vi "Test.vi"() -> ()   [LabVIEW 2015, in "SLSC Switch.lvlib" / "slscsl.lvclass"]
uses:
  slscsl.lvclass
  SwitchActionsArray.ctl
  SwitchAction.ctl
  RelayAction.ctl
panel:
  out "Relays":T1 {"RelayAction" items=["CloseRelay"=21, "OpenRelay"=20]}
  out "Disconnect":T1 {"RelayAction" items=["CloseRelay"=21, "OpenRelay"=20]}
  out "Connect":T1 {"RelayAction" items=["CloseRelay"=21, "OpenRelay"=20]}
  in  "error in (no error)":errorcluster
  out "error out":errorcluster
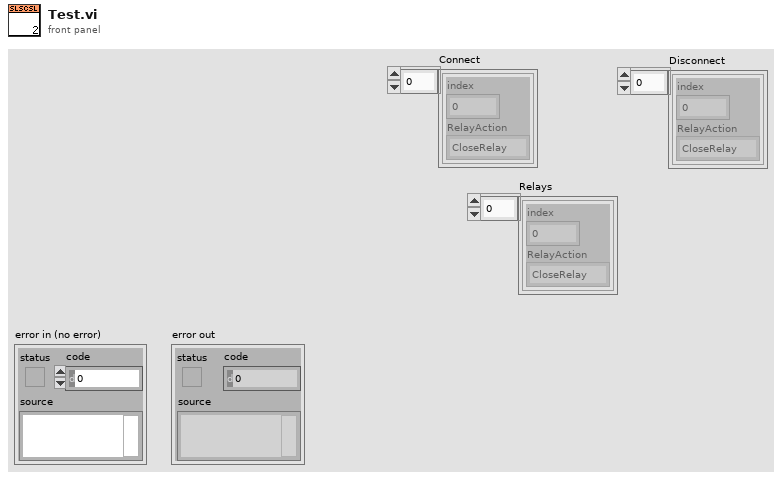
[diagram p1: front panel]
types:
  T1 = typedef "SLSC Switch.lvlib/slscsl.lvclass/SwitchActionsArray.ctl" = T2[]
  T2 = typedef "SLSC Switch.lvlib/slscsl.lvclass/SwitchAction.ctl" = cluster{"index":i32, "RelayAction":T3}
  T3 = typedef "SLSC Switch.lvlib/slscsl.lvclass/RelayAction.ctl" = u32
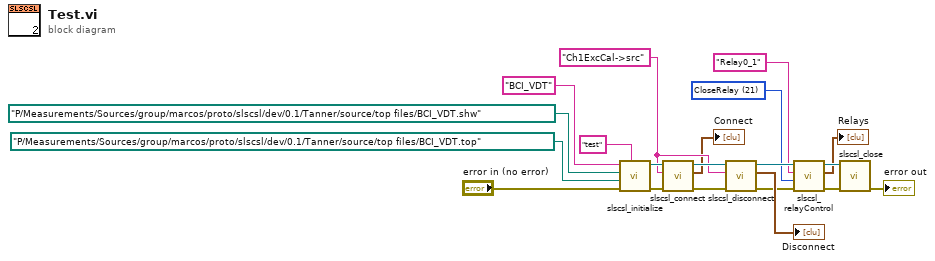
[diagram p0: block diagram]
diagram:
  w2 = T3 21 items=["CloseRelay"=21, "OpenRelay"=20] ("RelayAction")
  w10 = "Ch1ExcCal->src" ("channel 1")
  n1 = call "slscsl_initialize.vi"("deviceIdentifier"="test", "error in (no error)"="error in (no error)", "top file path"=path "P:/Measurements/Sources/group/marcos/proto/slscsl/dev/0.1/Tanner/source/top files/BCI_VDT.top", "shw file path"=path "P:/Measurements/Sources/group/marcos/proto/slscsl/dev/0.1/Tanner/source/top files/BCI_VDT.shw", "topologyName"="BCI_VDT") -> ("error out"=w13:errorcluster, "slscsl out"=w14:refnum<class "slscsl.lvclass">)  [unwired: 5 in]
  n2 = call "slscsl_connect.vi"("error in (no error)"=w13, "connectionList"=w10, "slscsl in"=w14) -> ("error out"=w11:errorcluster, "switchActionsArray"=→"Connect":T1, "slscsl out"=w12:refnum<class "slscsl.lvclass">)  [unwired: 6 in]
  n3 = call "slscsl_disconnect.vi"("error in (no error)"=w11, "connectionList"=w10, "slscsl in"=w12) -> ("error out"=w5:errorcluster, "SwitchActionsArray"=→"Disconnect":T1, "slscsl out"=w7:refnum<class "slscsl.lvclass">)  [unwired: 6 in]
  n4 = call "slscsl_relayControl.vi"("error in (no error)"=w5, "RelayAction"=w2, "relayNames"="Relay0_1", "slscsl in"=w7) -> ("error out"=w4:errorcluster, "switchActionArray"=→"Relays":T1, "slscsl out"=w6:refnum<class "slscsl.lvclass">)  [unwired: 5 in]
  n5 = call "slscsl_close.vi"("error in (no error)"=w4, "slscsl in"=w6) -> ("error out"=→"error out":errorcluster)  [unwired: 9 in]
